vi "new_P13.vi"(6 "Boolean":bool, 8 "E13":fxp<+,32,16>, 9 "P13":fxp<+,32,16>, 10 "feedback_time (ms)":fxp<+,16,1>, 11 "P33":fxp<+,32,16>) -> (2 "output valid":bool, 3 "P13 + dt*P33 + E13":fxp<+,32,16>)   [LabVIEW 2020]
uses:
  <vilib>/rvi/FXPMathLib/FxpMul/XNode/nifxpmath_Multiplier.xnode
  <vilib>/rvi/FXPMathLib/FxpAdd/XNode/nifxpmath_Add.xnode
  <vilib>/rvi/FXPMathLib/sim/FxpSim.dll
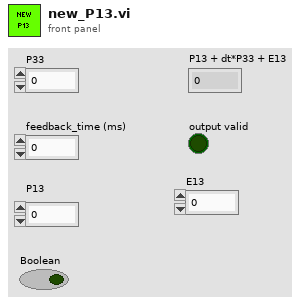
[diagram p1: front panel]
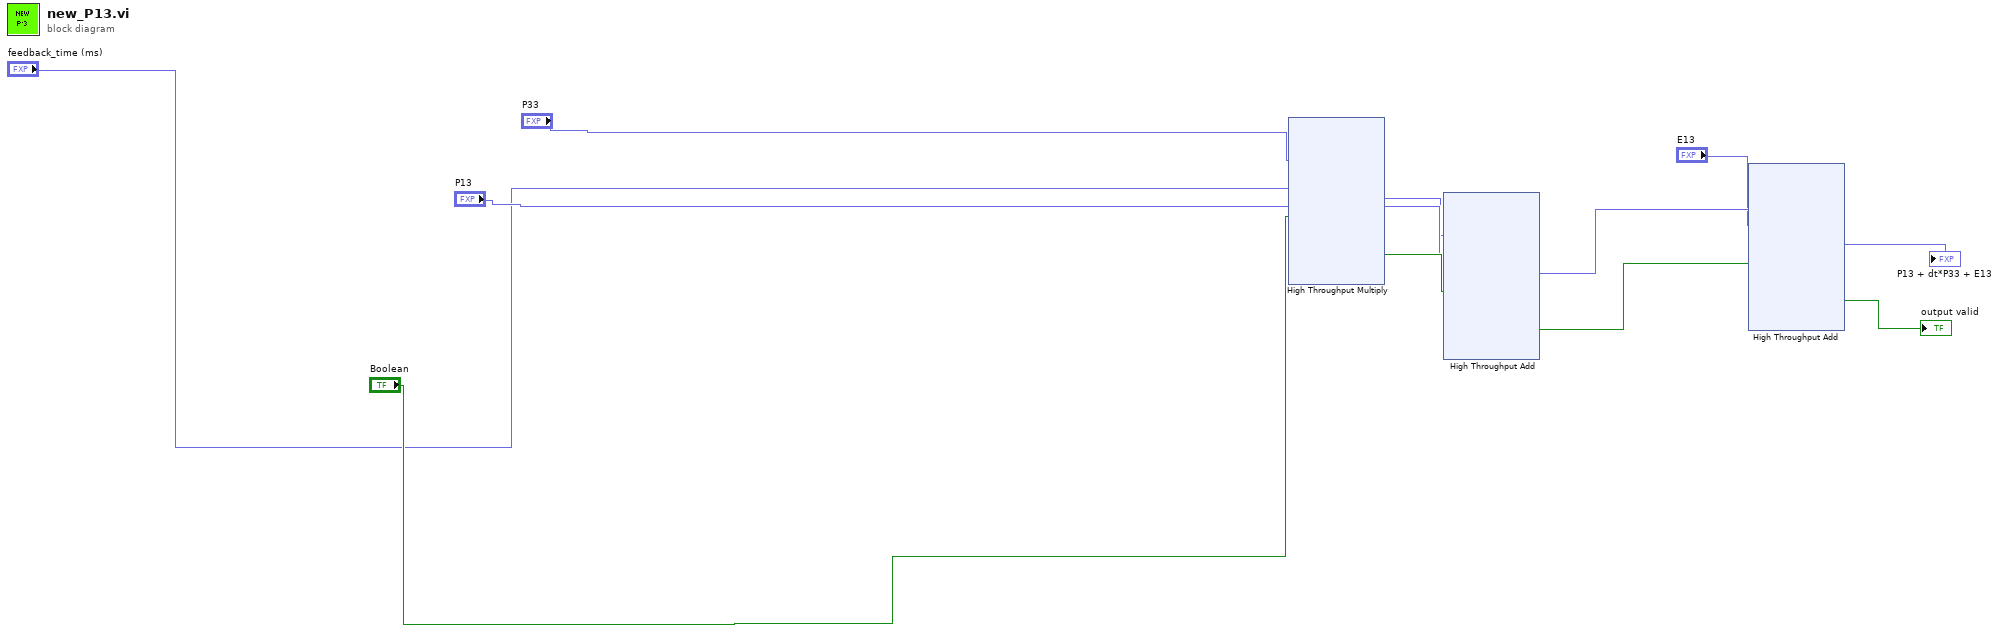
[diagram p0: block diagram]
diagram:
  n1 = xnode "High Throughput Multiply"("x"="P33", "y"="feedback_time (ms)", "input valid"="Boolean") -> ("x*y"=w8:fxp<+,48,17>, "output valid"=w11:bool)  [unwired: 1 in, 1 out]
  n2 = xnode "High Throughput Add"("x"=w8, "y"="P13", "input valid"=w11) -> ("x+y"=w5:fxp<+,32,16>, "output valid"=w3:bool)  [unwired: 1 in, 1 out]
  n3 = xnode "High Throughput Add"("x"=w5, "y"="E13", "input valid"=w3) -> ("x+y"=→"P13 + dt*P33 + E13":fxp<+,32,16>, "output valid"=→"output valid":bool)  [unwired: 1 in, 1 out]
